vi "Setup UI.vi"(8 "error in (no error)":errorcluster, 10 "Set UI to input? (F)":bool, 11 "Pulse Gen Basic Scan in":refnum<class "Pulse Gen Basic Scan.lvclass">) -> (0 "error out":errorcluster, 3 "Pulse Gen Basic Scan out":refnum<class "Pulse Gen Basic Scan.lvclass">)   [LabVIEW 2009, in "Pulse Gen Basic Scan.lvclass"]
doc: "Scanner::Setup is a constructor that has no parameters and faces the user. The Factory calls this VI to let the user configure this Scanner. It is dynamically dispatched in order to let the user choose the type as well as the options of the scanner."
uses:
  Pulse Gen Basic Scan.lvclass
  Pulse Gen Basic Scan.lvclass/Pulse Gen Basic Scan.ctl
panel:
  in  "Continuous Pulse/ \nExt Triggered Pulse":bool
  in  "Ch2 Width/Duty":bool=TRUE
  in  "Ch1 Width/Duty":bool=TRUE
  in  "Ch2 %Duty":dbl
  in  "Ch1 %Duty":dbl
  in  "Overall Frequency":dbl[unit]
  in  "period/frequency":bool
  in  "Send conds for first point to PG":bool
  in  "Ch2Width ind variable?":bool
  in  "Ch2Delay ind variable?":bool
  in  "Ch1Width ind variable?":bool
  in  "Ch1Delay ind variable?":bool
  in  "Ch2Width":dbl[unit]
  in  "Ch2Delay":dbl[unit]
  in  "Ch1Width":dbl[unit]
  in  "Ch1Delay":dbl[unit]
  in  "Overall Period":dbl[unit]
  # "Pulse Gen Basic Scan"
  # "Pulse Gen Basic Scan: This forces the PG to CONTINUOUS PULSES mode, and allowes the user to vary only the basic settings that could be changed from the front panel. \nNote: independent variable must be in ns."
  # "ind. variable?"
  # "Desired overall period/frequency"
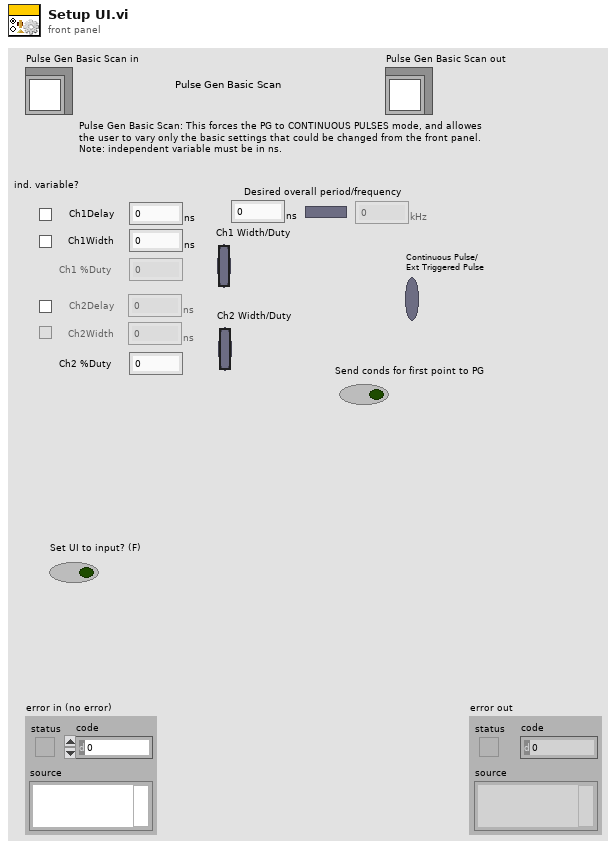
[diagram p1: front panel]
types:
  T1 = enum8{"Enabled", "Disabled", "Disabled and Grayed Out"}
  T2 = typedef "Scanner.lvclass/Range.ctl" = cluster{"xi":dbl, "xf":dbl, "dx":dbl, "Return to...?":bool, "Return to":dbl}
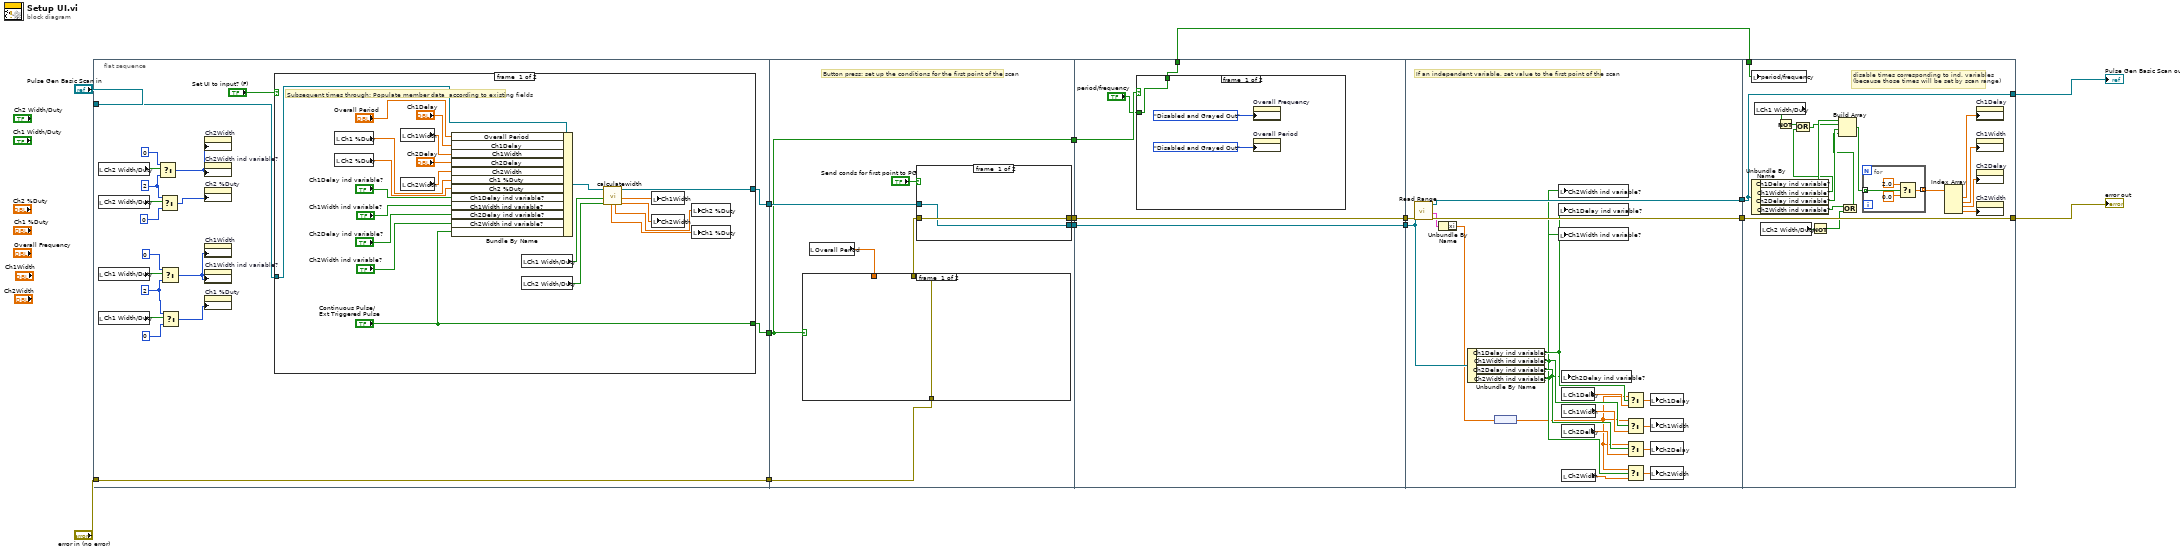
[diagram p0: block diagram]
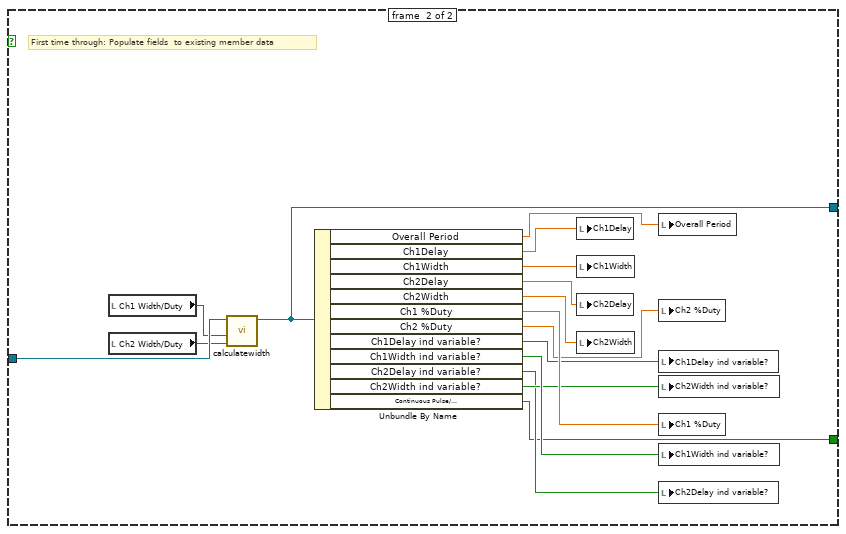
[diagram p2: hidden frame]
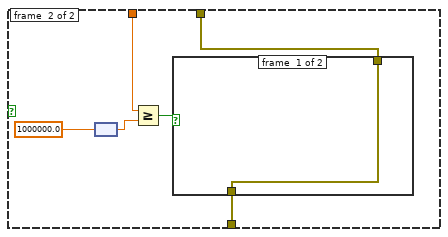
[diagram p3: hidden frame]
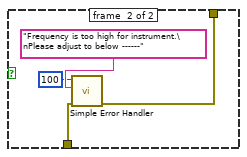
[diagram p4: hidden frame]
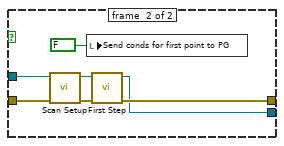
[diagram p5: hidden frame]
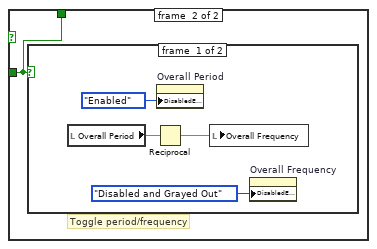
[diagram p6: hidden frame]
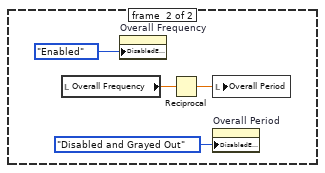
[diagram p7: hidden frame]
diagram:
  n1 = flat-sequence {
    tunnel: "error in (no error)" -> [w34]
    tunnel: "Pulse Gen Basic Scan in" -> [w33]
    tunnel: [w34] -> w12
    tunnel: [w17] -> w11
    tunnel: [w16] -> w2
    tunnel: w12 -> [w75]
    tunnel: w11 -> [w77]
    tunnel: [w78] -> w9
    tunnel: [w76] -> w8
    tunnel: w2 -> [w73]
    tunnel: [w73] -> w1
    tunnel: w9 -> [w105]
    tunnel: w8 -> [w103]
    tunnel: [w105] -> w7
    tunnel: [w103] -> w6
    tunnel: [w104] -> w3
    tunnel: w1 -> [w102]
    tunnel: w7 -> [w134]
    tunnel: w6 -> [w136]
    tunnel: [w133] -> w5
    tunnel: [w135] -> w4
    tunnel: [w149] -> w10
    tunnel: [w155] -> w15
    tunnel: w5 -> [w155]
    tunnel: w4 -> [w149]
    tunnel: w3 -> [w145]
    frame #0 {
      w23 = 2
      w20 = 2
      n2 = local read "Ch2 Width/Duty"() -> (w32:bool)
      n3 = local read "Ch2 Width/Duty"() -> (w29:bool)
      n4 = local read "Ch1 Width/Duty"() -> (w30:bool)
      n5 = local read "Ch1 Width/Duty"() -> (w31:bool)
      n6 = Select(t=0, s=w32, f=w23) -> (s? t:f=w24:i32)
      n7 = Select(t=w23, s=w29, f=0) -> (s? t:f=w22:i32)
      n8 = Select(t=0, s=w30, f=w20) -> (s? t:f=w21:i32)
      n9 = Select(t=w20, s=w31, f=0) -> (s? t:f=w19:i32)
      n10 = property on="Ch2Width" class="DigNum (strict)"("DisabledEnum"=w24) -> ()  [unwired: 2 in, 2 out]
      n11 = property on="Ch2Width ind variable?" class="Bool (strict)"("DisabledEnum"=w24) -> ()  [unwired: 2 in, 2 out]
      n12 = property on="Ch2 %Duty" class="DigNum (strict)"("DisabledEnum"=w22) -> ()  [unwired: 2 in, 2 out]
      n13 = property on="Ch1Width" class="DigNum (strict)"("DisabledEnum"=w21) -> ()  [unwired: 2 in, 2 out]
      n14 = property on="Ch1Width ind variable?" class="Bool (strict)"("DisabledEnum"=w21) -> ()  [unwired: 2 in, 2 out]
      n15 = property on="Ch1 %Duty" class="DigNum (strict)"("DisabledEnum"=w19) -> ()  [unwired: 2 in, 2 out]
      n16 = case shown="False" "Set UI to input? (F)" {
        tunnel: w33 -> [w50 w60]
        tunnel: [w44 w59] -> w17
        tunnel: ["Continuous Pulse/ \nExt Triggered Pulse" w56] -> w16
        frame #0 {
          # "Subsequent times through: Populate member data  according to existing fields"
          n17 = local read "Ch1 %Duty"() -> (w47:dbl)
          n18 = local read "Ch2 %Duty"() -> (w46:dbl)
          n19 = local read "Ch1Width"() -> (w49:dbl[unit])
          n20 = local read "Ch2Width"() -> (w48:dbl[unit])
          n21 = Bundle By Name(cluster=w50, "Overall Period"="Overall Period", "Ch1Delay"="Ch1Delay", "Ch1Width"=w49, "Ch2Delay"="Ch2Delay", "Ch2Width"=w48, "Ch1 %Duty"=w47, "Ch2 %Duty"=w46, "Ch1Delay ind variable?"="Ch1Delay ind variable?", "Ch1Width ind variable?"="Ch1Width ind variable?", "Ch2Delay ind variable?"="Ch2Delay ind variable?", "Ch2Width ind variable?"="Ch2Width ind variable?", "Continuous Pulse/ \nExt Triggered Pulse"="Continuous Pulse/ \nExt Triggered Pulse") -> (w45:refnum<class "Pulse Gen Basic Scan.lvclass">)
          n22 = local read "Ch1 Width/Duty"() -> (w43:bool)
          n23 = local read "Ch2 Width/Duty"() -> (w42:bool)
          n24 = call "calculatewidth.vi"("Ch2 Width/Duty"=w42, "Ch1 Width/Duty"=w43, "Pulse Gen Basic Scan.lvclass"=w45) -> ("Ch2 Width"=w40:dbl[unit], "Ch1 Width"=w41:dbl[unit], "Pulse Gen Basic Scan.lvclass 2"=w44:refnum<class "Pulse Gen Basic Scan.lvclass">, "Ch2 %Duty"=w38:dbl, "Ch1 %Duty"=w39:dbl)  [unwired: 4 in]
          n25 = local write "Ch1Width"(w41) -> ()
          n26 = local write "Ch2Width"(w40) -> ()
          n27 = local write "Ch2 %Duty"(w38) -> ()
          n28 = local write "Ch1 %Duty"(w39) -> ()
        }
        frame #1 {
          # "First time through: Populate fields  to existing member data"
          n29 = local read "Ch1 Width/Duty"() -> (w58:bool)
          n30 = local read "Ch2 Width/Duty"() -> (w57:bool)
          n31 = call "calculatewidth.vi"("Ch2 Width/Duty"=w57, "Ch1 Width/Duty"=w58, "Pulse Gen Basic Scan.lvclass"=w60) -> ("Pulse Gen Basic Scan.lvclass 2"=w59:refnum<class "Pulse Gen Basic Scan.lvclass">)  [unwired: 4 in, 4 out]
          n32 = Unbundle By Name(w59) -> ("Overall Period"=w71:dbl[unit], "Ch1Delay"=w69:dbl[unit], "Ch1Width"=w70:dbl[unit], "Ch2Delay"=w68:dbl[unit], "Ch2Width"=w67:dbl[unit], "Ch1 %Duty"=w66:dbl, "Ch2 %Duty"=w61:dbl, "Ch1Delay ind variable?"=w65:bool, "Ch1Width ind variable?"=w64:bool, "Ch2Delay ind variable?"=w62:bool, "Ch2Width ind variable?"=w63:bool, "Continuous Pulse/ \nExt Triggered Pulse"=w56:bool)
          n33 = local write "Ch1Delay"(w69) -> ()
          n34 = local write "Ch1Width"(w70) -> ()
          n35 = local write "Ch2Delay"(w68) -> ()
          n36 = local write "Ch2Width"(w67) -> ()
          n37 = local write "Overall Period"(w71) -> ()
          n38 = local write "Ch2 %Duty"(w61) -> ()
          n39 = local write "Ch1Delay ind variable?"(w65) -> ()
          n40 = local write "Ch2Width ind variable?"(w63) -> ()
          n41 = local write "Ch1 %Duty"(w66) -> ()
          n42 = local write "Ch1Width ind variable?"(w64) -> ()
          n43 = local write "Ch2Delay ind variable?"(w62) -> ()
        }
      }
    }
    frame #1 {
      # "Button press: set up the conditions for the first point of the scan"
      n44 = local read "Overall Period"() -> (w72:dbl[unit])
      n45 = case shown="False" w73 {
        tunnel: w75 -> [w80 w86]
        tunnel: [w80 w85] -> w74
        tunnel: w72 -> [_ w81]
        frame #0 {
        }
        frame #1 {
          n46 = node(1000000.0 ("y")) -> (w83:dbl[unit])
          n47 = Greater Or Equal?(x=w81, y=w83) -> (x >= y?=w82:bool)
          n48 = case shown="True" w82 {
            tunnel: w86 -> [w87 w91]
            tunnel: [w87 w89] -> w85
            frame #0 {
            }
            frame #1 {
              n49 = call <vilib>:"Simple Error Handler.vi"("error code (no error:0)"=100, "error source (\" \")"="Frequency is too high for instrument.\nPlease adjust to below ------", "error in (no error)"=w91) -> ("error out"=w89:errorcluster)  [unwired: 2 in, 4 out]
            }
          }
        }
      }
      n50 = case shown="True" "Send conds for first point to PG" {
        tunnel: w74 -> [w93 w99]
        tunnel: [w93 w97] -> w78
        tunnel: w77 -> [w92 w96]
        tunnel: [w92 w94] -> w76
        frame #0 {
        }
        frame #1 {
          n51 = call-dynamic "Scan Setup.vi"("error in (no error)"=w99, "Pulse Gen Basic Scan in"=w96) -> ("error out"=w98:errorcluster, "Pulse Gen Basic Scan out"=w95:refnum<class "Pulse Gen Basic Scan.lvclass">)  [unwired: 8 in]
          n52 = local write "Send conds for first point to PG"(FALSE ("Send conds for first point to PG")) -> ()
          n53 = call-dynamic "First Step.vi"("error in (no error)"=w98, "Pulse Gen Basic Scan.lvclass in"=w95) -> ("error out"=w97:errorcluster, "Pulse Gen Basic Scan.lvclass out"=w94:refnum<class "Pulse Gen Basic Scan.lvclass">)  [unwired: 7 in, 1 out]
        }
      }
    }
    frame #2 {
      n54 = case shown="False" w102 {
        tunnel: [w106 w109] -> w104
        tunnel: "period/frequency" -> [w106 w109]
        frame #0 {
          n55 = property on="Overall Frequency" class="DigNum (strict)"("DisabledEnum"=T1."Disabled and Grayed Out" ("Disabled")) -> ()  [unwired: 2 in, 2 out]
          n56 = property on="Overall Period" class="DigNum (strict)"("DisabledEnum"=T1."Disabled and Grayed Out" ("Disabled")) -> ()  [unwired: 2 in, 2 out]
        }
        frame #1 {
          # "Toggle period/frequency"
          n57 = case shown="True" w109 {
            frame #0 {
              n58 = local read "Overall Period"() -> (w113:dbl[unit])
              n59 = Reciprocal(x=w113) -> (1/x=w112:dbl[unit])
              n60 = property on="Overall Period" class="DigNum (strict)"("DisabledEnum"=T1."Enabled" ("Disabled")) -> ()  [unwired: 2 in, 2 out]
              n61 = local write "Overall Frequency"(w112) -> ()
              n62 = property on="Overall Frequency" class="DigNum (strict)"("DisabledEnum"=T1."Disabled and Grayed Out" ("Disabled")) -> ()  [unwired: 2 in, 2 out]
            }
            frame #1 {
              n63 = local read "Overall Frequency"() -> (w115:dbl[unit])
              n64 = property on="Overall Frequency" class="DigNum (strict)"("DisabledEnum"=T1."Enabled" ("Disabled")) -> ()  [unwired: 2 in, 2 out]
              n65 = Reciprocal(x=w115) -> (1/x=w114:dbl[unit])
              n66 = local write "Overall Period"(w114) -> ()
              n67 = property on="Overall Period" class="DigNum (strict)"("DisabledEnum"=T1."Disabled and Grayed Out" ("Disabled")) -> ()  [unwired: 2 in, 2 out]
            }
          }
        }
      }
    }
    frame #3 {
      # "If an independent variable, set value to the first point of the scan"
      n68 = call-dynamic "Read Range.vi"("error in (no error)"=w134, "Scanner.lvclass in"=w136) -> ("error out"=w133:errorcluster, "Range"=w132:T2, "Scanner.lvclass out"=w135:refnum<class "Pulse Gen Basic Scan.lvclass">)  [unwired: 7 out]
      n69 = Unbundle By Name(w132) -> ("xi"=w119:dbl)
      n70 = Unbundle By Name(w136) -> ("Ch1Delay ind variable?"=w123:bool, "Ch1Width ind variable?"=w122:bool, "Ch2Delay ind variable?"=w121:bool, "Ch2Width ind variable?"=w120:bool)
      n71 = node(w119) -> (w118:dbl[unit])
      n72 = local write "Ch2Width ind variable?"(w120) -> ()
      n73 = local write "Ch1Delay ind variable?"(w123) -> ()
      n74 = local write "Ch1Width ind variable?"(w122) -> ()
      n75 = local write "Ch2Delay ind variable?"(w121) -> ()
      n76 = local read "Ch1Delay"() -> (w124:dbl[unit])
      n77 = local read "Ch1Width"() -> (w125:dbl[unit])
      n78 = local read "Ch2Delay"() -> (w126:dbl[unit])
      n79 = local read "Ch2Width"() -> (w127:dbl[unit])
      n80 = Select(t=w118, s=w123, f=w124) -> (s? t:f=w131:dbl[unit])
      n81 = Select(t=w118, s=w122, f=w125) -> (s? t:f=w130:dbl[unit])
      n82 = Select(t=w118, s=w121, f=w126) -> (s? t:f=w129:dbl[unit])
      n83 = Select(t=w118, s=w120, f=w127) -> (s? t:f=w128:dbl[unit])
      n84 = local write "Ch1Delay"(w131) -> ()
      n85 = local write "Ch1Width"(w130) -> ()
      n86 = local write "Ch2Delay"(w129) -> ()
      n87 = local write "Ch2Width"(w128) -> ()
    }
    frame #4 {
      # "disable times corresponding to ind. variables \n(because those times will be set by scan range)"
      n88 = Unbundle By Name(w149) -> ("Ch1Delay ind variable?"=w148:bool, "Ch1Width ind variable?"=w142:bool, "Ch2Delay ind variable?"=w147:bool, "Ch2Width ind variable?"=w138:bool)
      n89 = local write "period/frequency"(w145) -> ()
      n90 = local read "Ch1 Width/Duty"() -> (w144:bool)
      n91 = local read "Ch2 Width/Duty"() -> (w140:bool)
      n92 = Not(x=w144) -> (.not. x?=w143:bool)
      n93 = Or(x=w143, y=w142) -> (x .or. y?=w141:bool)
      n94 = Not(x=w140) -> (.not. x?=w139:bool)
      n95 = Or(x=w138, y=w139) -> (x .or. y?=w137:bool)
      n96 = Build Array(w148, w141, w147, w137) -> (w146:bool[])
      n97 = for {
        tunnel: [w157] -> w154 mode=indexing
        tunnel: w146 -> [w156] mode=indexing
        n98 = Select(t=2.0, s=w156, f=0.0) -> (s? t:f=w157:dbl)
      }
      n99 = Index Array(array=w154) -> (element #1=w153:dbl, element #2=w152:dbl, element #3=w151:dbl, element #4=w150:dbl)  [unwired: 4 in]
      n100 = property on="Ch1Delay" class="DigNum (strict)"("DisabledEnum"=w153) -> ()  [unwired: 2 in, 2 out]
      n101 = property on="Ch1Width" class="DigNum (strict)"("DisabledEnum"=w152) -> ()  [unwired: 2 in, 2 out]
      n102 = property on="Ch2Delay" class="DigNum (strict)"("DisabledEnum"=w151) -> ()  [unwired: 2 in, 2 out]
      n103 = property on="Ch2Width" class="DigNum (strict)"("DisabledEnum"=w150) -> ()  [unwired: 2 in, 2 out]
    }
  }
  "error out" <- w15
  "Pulse Gen Basic Scan out" <- w10
